vi "TOF spectrum.vi"() -> ()   [LabVIEW 2021]
uses:
  <userlib>/SciSDK/SciSDK_Labview.lvlib
panel:
  out "data":i32[](array[numeric])
  out "Valid Bins":u32
  out "Total Bins":u32
  out "Buffer Size":u32
  out "Integration time":u32
  out "Timecode":u32
  out "Magic":u32
  out "Histogram":i32[](graph)
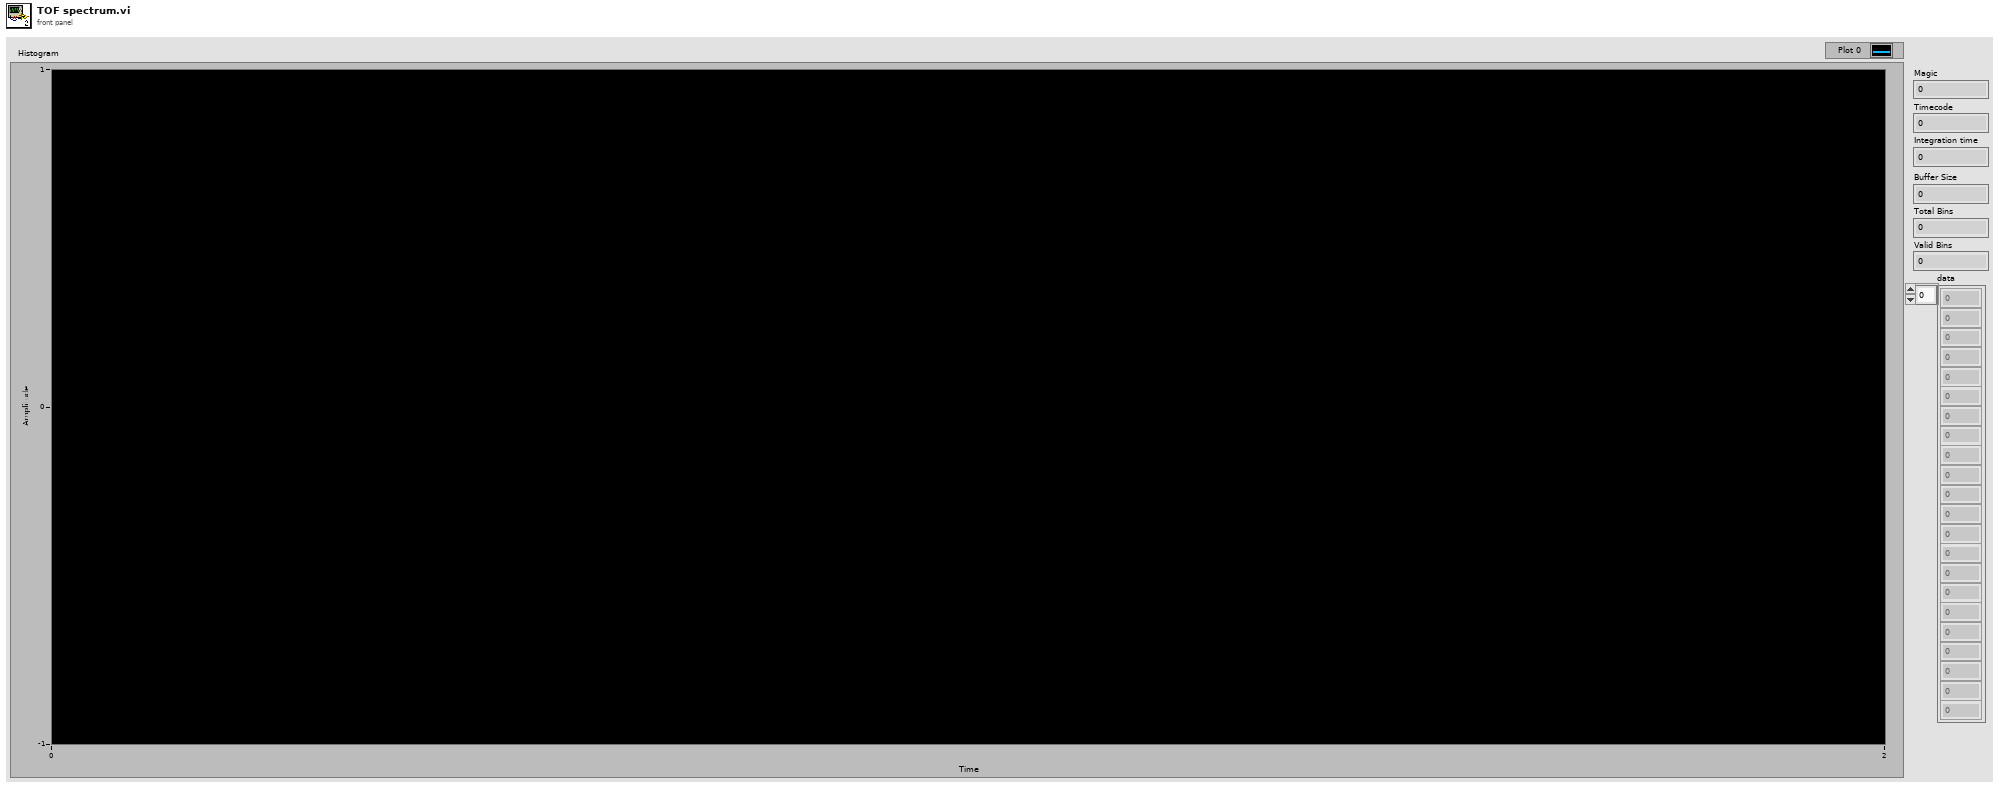
[diagram p1: front panel]
types:
  T1 = cluster{"Name":string, "Board Model":string, "Handle":u64}
  T2 = cluster{"TOF Spectrum Path":string, "TOF Spectrum Name":string}
  T3 = cluster{"Board Name":string, "Board Model":string, "Handle":u64}
  T4 = cluster{"magic":u32, "timecode":u32, "inttime":u32, "buffer_size":u32, "total_bins":u32, "valid_bins":u32, "data":i32[]}
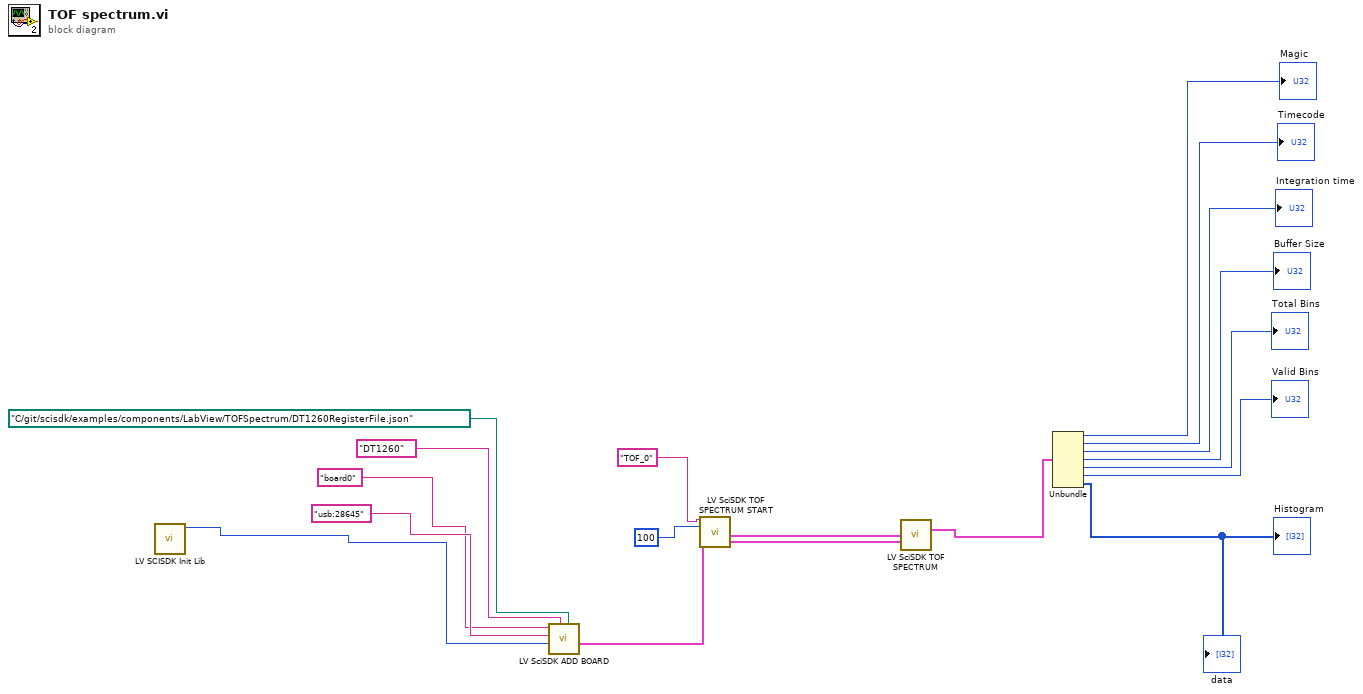
[diagram p0: block diagram]
diagram:
  n1 = call <userlib>:"LV SCISDK Init Lib.vi"() -> ("function return"=w11:u64)  [unwired: 11 in]
  n2 = call <userlib>:"LV SciSDK ADD BOARD.vi"("JsonFile"=path "C:/git/scisdk/examples/components/LabView/TOFSpectrum/DT1260RegisterFile.json", "Board Model"="DT1260", "SciSDK Handle"=w11, "DevicePath"="usb:28645", "Name"="board0") -> ("Board Handle Out"=w6:T1)  [unwired: 4 in, 2 out]
  n3 = call <userlib>:"LV SciSDK TOF SPECTRUM START.vi"("TOF Spectrum Name"="TOF_0" ("Spectrum name"), "Bin Width"=u32 100, "Board Handle In"=w6) -> ("TOF Spectrum Handle Out"=w2:T2, "Board Handle Out"=w1:T3)  [unwired: 10 in, 1 out]
  n4 = call <userlib>:"LV SciSDK TOF SPECTRUM.vi"("TOF Spectrum Handle In"=w2, "Board Handle In"=w1) -> ("TOF Spectrum Buffer Out"=w3:T4)  [unwired: 9 in, 4 out]
  n5 = Unbundle(w3) -> ("magic"=→"Magic":u32, "timecode"=→"Timecode":u32, "inttime"=→"Integration time":u32, "buffer_size"=→"Buffer Size":u32, "total_bins"=→"Total Bins":u32, "valid_bins"=→"Valid Bins":u32, "data"=→"Histogram" →"data":i32[])
